vi "Practica04.vi"() -> ()   [LabVIEW 2020]
panel:
  out "Valor Mínimo":dbl
  out "Valor Máximo":dbl
  in  "stop":bool
  out "Waveform Chart":dynamicdata(graph)
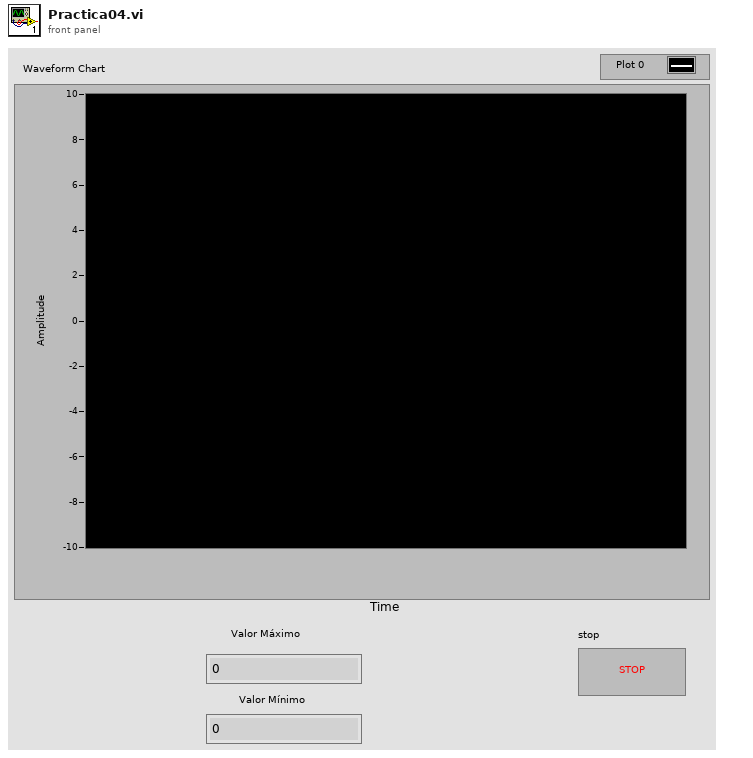
[diagram p1: front panel]
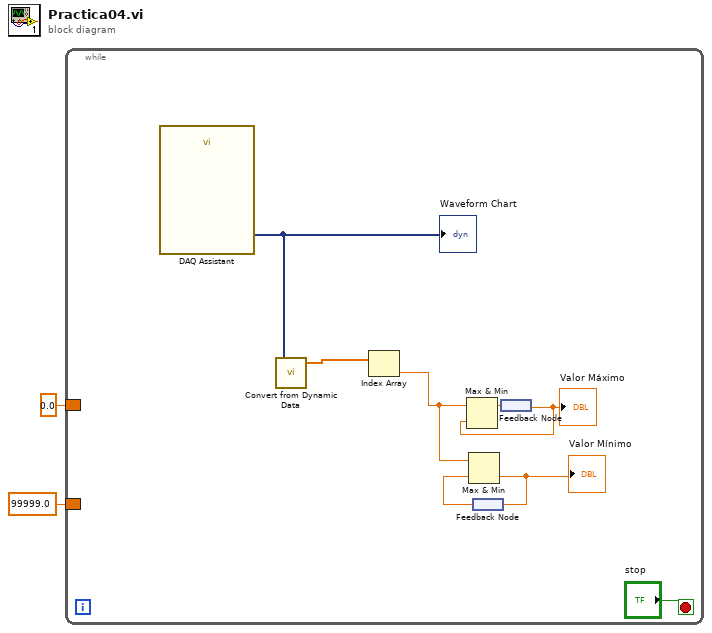
[diagram p0: block diagram]
diagram:
  n1 = while {
    border: 0.0 -> [_]
    border: 99999.0 -> [_]
    stop <- "stop" stop-if-true
    n2 = call "DAQ Assistant"() -> ("data"=w10:dynamicdata)  [unwired: 17 in, 2 out]
    "Waveform Chart" <- w10
    n3 = call "Convert from Dynamic Data"("Dynamic Data Type"=w10) -> ("Array"=w9:dbl[])  [unwired: 3 in]
    n4 = Index Array "Index Array"(array=w9) -> (element=w5:dbl)  [unwired: 1 in]
    n5 = feedback #1() -> (w3:dbl)
    n6 = Max & Min(x=w5, y=w3) -> (min(x,y)=w4:dbl)  [unwired: 1 out]
    "Valor Mínimo" <- w4
    n7 = feedback-in #1(w4) -> ()
    n8 = feedback #2() -> (w6:dbl)
    "Valor Máximo" <- w6
    n9 = Max & Min(x=w5, y=w6) -> (max(x,y)=w7:dbl)  [unwired: 1 out]
    n10 = feedback-in #2(w7) -> ()
  }
